vi "Solve_Problems_Tracks_NN-1.vi"(0 "Tracks (unsorted, cols)":dbl[][](array[numeric]), 1 "Max angle":dbl min=1.0 max=90.0 step=1.0, 2 "X,Y":dbl[][](array[numeric]), 3 "error IN":errorcluster, 4 "Areas":dbl[][](array[numeric])) -> (5 "Tracks (X,Y,dX,dY)":dbl[][](array[numeric]), 6 "# of Found \ndisplacements":i32, 7 "error OUT":errorcluster)   [LabVIEW 2013]
doc: "Top-level subVI performs Nearest Neighbor algorithm for tracking (for comparing of tracking results)"
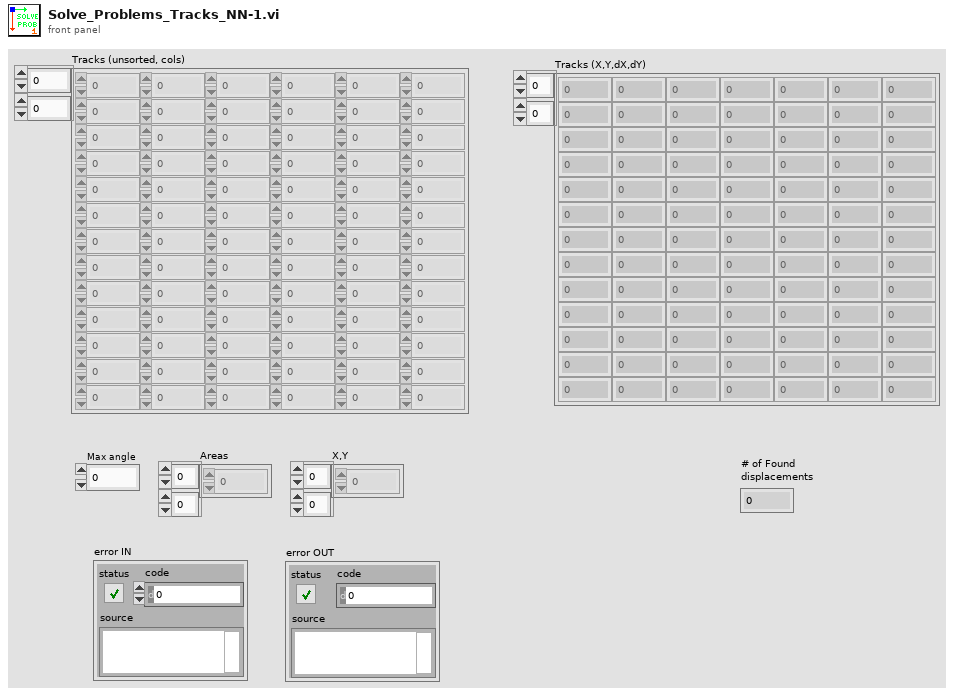
[diagram p1: front panel]
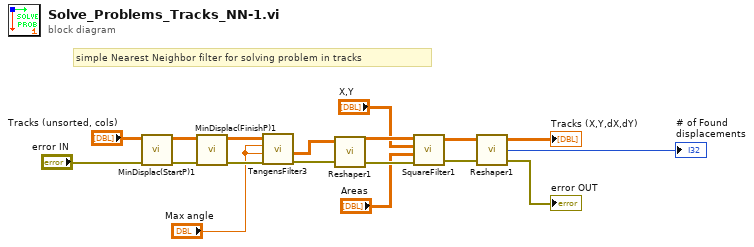
[diagram p0: block diagram]
diagram:
  # "simple Nearest Neighbor filter for solving problem in tracks"
  n1 = call "MinDisplac(StartP)1.vi"("error IN"="error IN", "IN (X,Y,dX,dY) NN"="Tracks (unsorted, cols)") -> ("error OUT"=w17:errorcluster, "OUT (X,Y,dX,dY) MINIMAL"=w18:dbl[][])  [unwired: 3 in, 1 out]
  n2 = call "MinDisplac(FinishP)1.vi"("error IN"=w17, "IN (X,Y,dX,dY)"=w18) -> ("error OUT"=w12:errorcluster, "OUT (X,Y,dX,dY) MINIMAL"=w11:dbl[][])  [unwired: 3 in, 1 out]
  n3 = call "TangensFilter3.vi"("error IN"=w12, "Max Angle REVERSE Disp"="Max angle", "Max Angle FORWARD Displ"="Max angle", "Finded Chains (X,Y,dX,dY)"=w11) -> ("error out"=w10:errorcluster, "Filtered Chains (X,Y,dX,dY)"=w9:dbl[][])  [unwired: 2 out]
  n4 = call "Reshaper1.vi"("error IN"=w10, "[IN] (X,Y,dX,dY)"=w9) -> ("error OUT"=w15:errorcluster, "[OUT] Reshaped (X,Y,dX,dY)"=w16:dbl[][])  [unwired: 1 in, 1 out]
  n5 = call "SquareFilter1.vi"("error IN"=w15, "Areas"="Areas", "X,Y"="X,Y", "Chains (X,Y,dX,dY)"=w16) -> ("error OUT"=w13:errorcluster, "Filtered Chains (X,Y,dX,dY)"=w14:dbl[][])  [unwired: 1 out]
  n6 = call "Reshaper1.vi"("error IN"=w13, "[IN] (X,Y,dX,dY)"=w14) -> ("error OUT"=→"error OUT":errorcluster, "Numeric"=→"# of Found \ndisplacements":i32, "[OUT] Reshaped (X,Y,dX,dY)"=→"Tracks (X,Y,dX,dY)":dbl[][])  [unwired: 1 in]
